vi "HCCConfig.vi"() -> ()   [LabVIEW 2014]
uses:
  c_MicroZedInstr_Enum.ctl
  g_ReportControl.vi
  <vilib>/Utility/file.llb/Read From Spreadsheet File (string).vi
  g_HCCRegisterConfig.vi
  <vilib>/Utility/file.llb/Write To Spreadsheet File (string).vi
  g_MicroZed_Interface.vi
  g_Stop.vi
  <vilib>/regexp/Match Regular Expression.xnode
panel:
  out "Transmission Error":bool
  in  "Register":T1(ring)
  in  "Write Register":bool
  in  "Value":string=" 0x00000000"
  in  "OK":bool
  out "Table":string[][](table)=[["HCC Register", "Address", "Value", "Default Values"], ["HCC_REG_0", " 0x00", "", " 0x0007FEC5"], ["HCC_REG_1", " 0x01", "", " 0xE0018080"], ["HCC_REG_2", " 0x02", "", " 0x00000840"], ["HCC_REG_3", " 0x03", "", " 0x000FFC00"], ["HCC_REG_4", " 0x04", "", " 0x3FF003FF"], ["HCC_REG_5", " 0x05", "", " 0x000FFC00"], ["HCC_REG_6", " 0x06", "", " 0x3FF003FF"], ["HCC_REG_7", " 0x07", "", " 0x000FFC00"], ["HCC_REG_8", " 0x08", "", " 0x00000000"], ["HCC_REG_9", " 0x09", "", " 0x39CE739C"], ["HCC_REG_10", " 0x10", "", " 0x00333304"], ["HCC_REG_11", " 0x11", "", " 0x01050402"], ["HCC_REG_12", " 0x12", "", " 0x00000000"], ["HCC_REG_13", " 0x13", "", " 0x00700000"], ["HCC_REG_14", " 0x14", "", " 0xFFF107FF"], ["HCC_REG_15", " 0x15", "", " 0xFFFFFFFF"], ["HCC_REG_16", " 0x16", "", " 0x00000000"], ["HCC_REG_17", " 0x17", "", " 0x00000000"]]
  in  "Store Custom":bool
  in  "Load Default":bool
  in  "Load Config File":bool
  # "HCC Register Configuration"
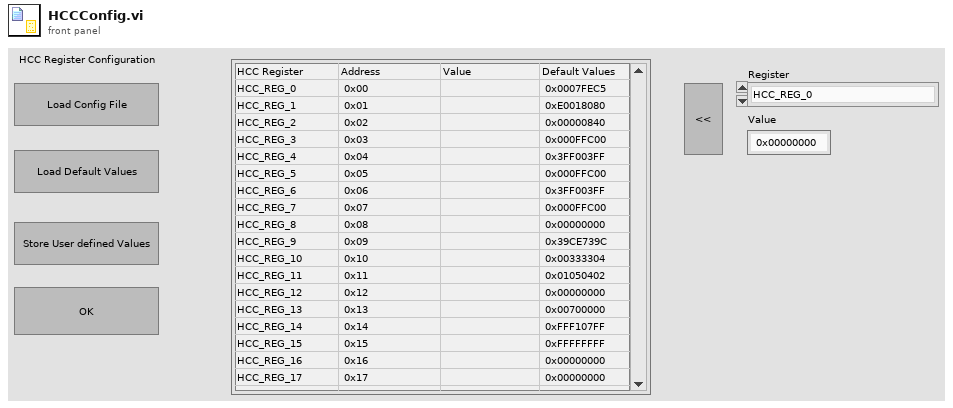
[diagram p1: front panel]
types:
  T1 = enum16{"HCC_REG_0", "HCC_REG_1", "HCC_REG_2", "HCC_REG_3", "HCC_REG_4", "HCC_REG_5", "HCC_REG_6", "HCC_REG_7", "HCC_REG_8", "HCC_REG_9", "HCC_REG_10", "HCC_REG_11", "HCC_REG_12", "HCC_REG_13", "HCC_REG_14", "HCC_REG_15", "HCC_REG_16", "HCC_REG_17"}
  T2 = typedef "c_MicroZedInstr_Enum.ctl" = enum16{"Start Test Procedure", "Print Instructions", "Config HCC Register", "Send Parameters"}
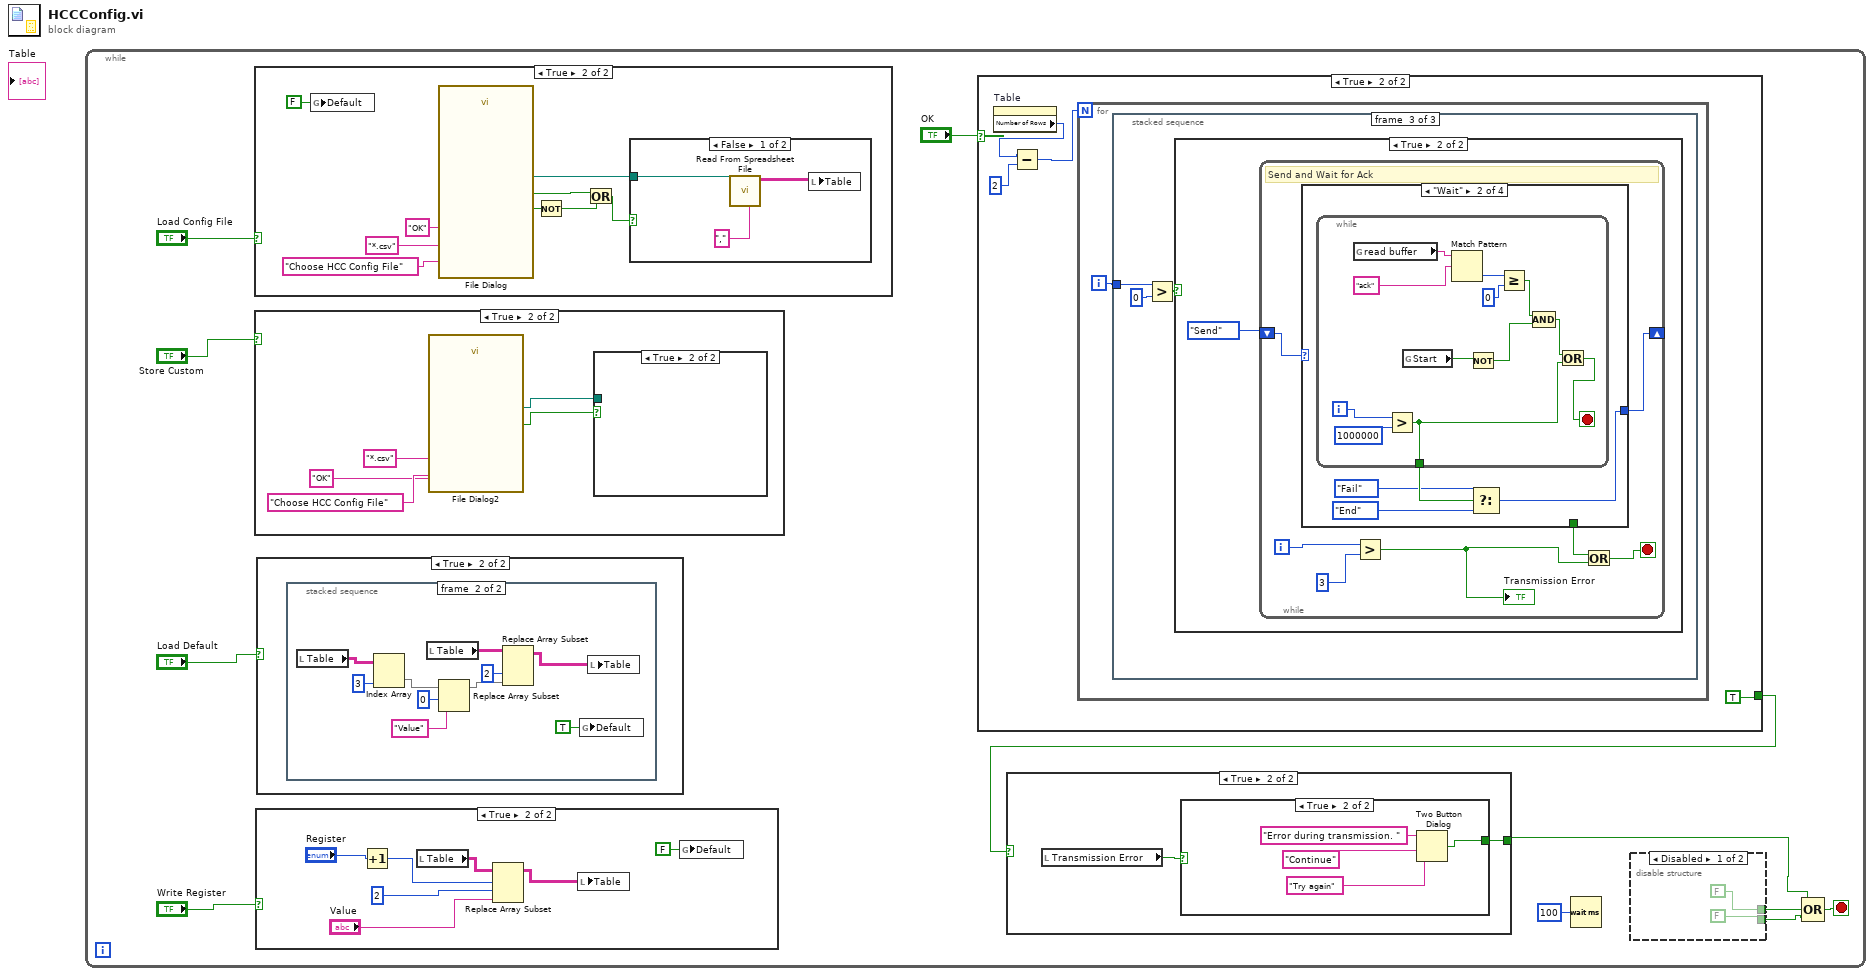
[diagram p0: block diagram]
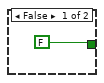
[diagram p2: hidden frame]
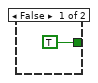
[diagram p3: hidden frame]
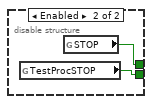
[diagram p4: hidden frame]
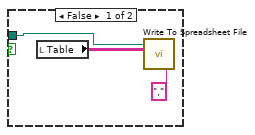
[diagram p6: hidden frame]
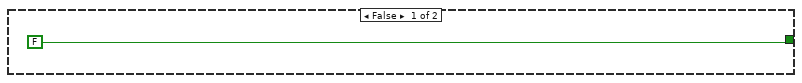
[diagram p8: hidden frame]
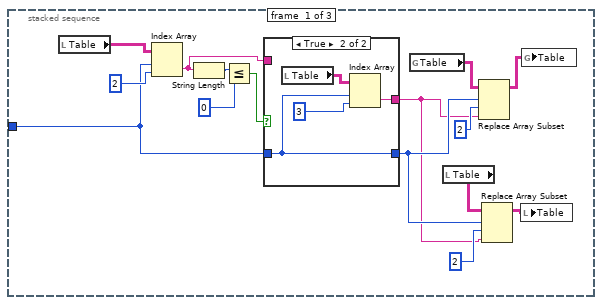
[diagram p9: hidden frame]
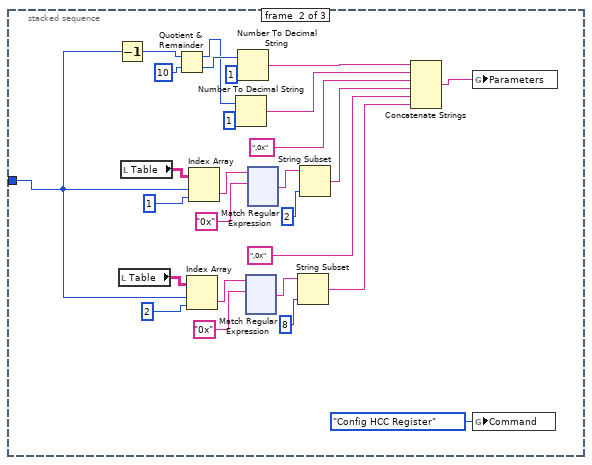
[diagram p11: hidden frame]
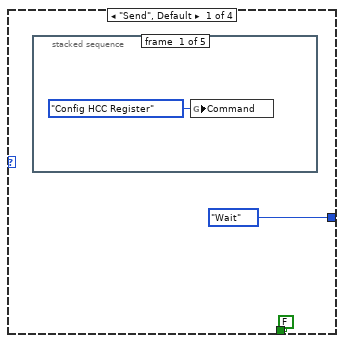
[diagram p13: hidden frame]
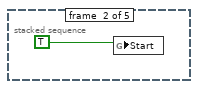
[diagram p14: hidden frame]
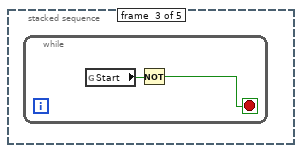
[diagram p15: hidden frame]
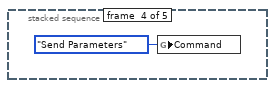
[diagram p16: hidden frame]
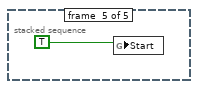
[diagram p17: hidden frame]
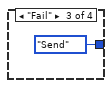
[diagram p18: hidden frame]
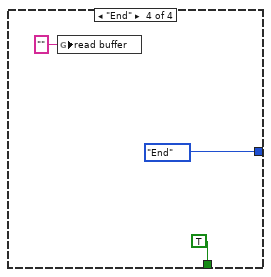
[diagram p19: hidden frame]
diagram:
  n1 = while {
    stop <- w5 stop-if-true
    n2 = case shown="True" "Load Config File" {
      frame False {
        n3 = global write "g_ReportControl.vi" "New Report"(FALSE ("New Report")) -> ()
      }
      frame True {
        n4 = global write "g_HCCRegisterConfig.vi" "Default"(FALSE ("Default")) -> ()
        n5 = call "File Dialog"("prompt"="Choose HCC Config File", "button label"="OK", "pattern (all files)"="*.csv") -> ("selected path"=w373:path, "exists"=w377:bool, "cancelled"=w375:bool)  [unwired: 9 in, 1 out]
        n6 = Not(x=w377) -> (.not. x?=w376:bool)
        n7 = Or(x=w375, y=w376) -> (x .or. y?=w374:bool)
        n8 = case shown="False" w374 {
          tunnel: w373 -> [w383 _]
          frame False {
            n9 = call-poly <vilib>:"Read From Spreadsheet File.vi"("delimiter (\\t)"="," ("delimiter (\\t)"), "file path (dialog if empty)"=w383) -> ("all rows"=w381:string[][])  [unwired: 5 in, 4 out]
            n10 = local write "Table"(w381) -> ()
          }
          frame True {
            n11 = One Button Dialog(message="Config File could not be loaded") -> ()  [unwired: 1 in, 1 out]
          }
        }
      }
    }
    n12 = case shown="True" "Store Custom" {
      frame False {
      }
      frame True {
        n13 = call "File Dialog2"("prompt"="Choose HCC Config File", "button label"="OK", "pattern (all files)"="*.csv") -> ("selected path"=w25:path, "cancelled"=w24:bool)  [unwired: 9 in, 2 out]
        n14 = case shown="True" w24 {
          tunnel: w25 -> [w29 _]
          frame False {
            n15 = local read "Table"() -> (w30:string[][])
            n16 = call-poly <vilib>:"Write To Spreadsheet File.vi"("delimiter (\\t)"="," ("delimiter (\\t)"), "2D data"=w30, "file path (dialog if empty)"=w29) -> ()  [unwired: 5 in, 1 out]
          }
          frame True {
          }
        }
      }
    }
    n17 = case shown="True" "Write Register" {
      frame False {
      }
      frame True {
        n18 = Increment(x="Register") -> (x+1=w33:T1)
        n19 = local read "Table"() -> (w37:string[][])
        n20 = Replace Array Subset(array=w37, new element="Value", index (row)=w33, index (col)=2 ("disabled index (col)")) -> (w38:string[][])
        n21 = local write "Table"(w38) -> ()
        n22 = global write "g_HCCRegisterConfig.vi" "Default"(FALSE ("Default")) -> ()
      }
    }
    n23 = case shown="True" "Load Default" {
      frame False {
      }
      frame True {
        n24 = stacked-sequence {
          frame #0 {
            n25 = control-ref of="Table"() -> (w360:refnum<vi>)
            n26 = invoke class="Tbl (strict)" method="Reinit To Default"(reference=w360) -> ()  [unwired: 2 in, 3 out]
          }
          frame #1 {
            n27 = local read "Table"() -> (w370:string[][])
            n28 = Index Array(array=w370, index (col)=3 ("disabled index (col)")) -> (element=w368:string[])  [unwired: 1 in]
            n29 = local read "Table"() -> (w364:string[][])
            n30 = Replace Array Subset(array=w368, new element="Value" ("new element/subarray"), index=0) -> (w365:string[])
            n31 = Replace Array Subset(array=w364, new element=w365, index (col)=2 ("disabled index (col)")) -> (w362:string[][])  [unwired: 1 in]
            n32 = global write "g_HCCRegisterConfig.vi" "Default"(TRUE ("Default")) -> ()
            n33 = local write "Table"(w362) -> ()
          }
        }
      }
    }
    n34 = case shown="True" "OK" {
      tunnel: [FALSE TRUE] -> w2
      frame False {
      }
      frame True {
        n35 = property on="Table" class="Tbl (strict)"() -> ("Number of Rows"=w42:u32)  [unwired: 2 in, 2 out]
        n36 = Subtract(x=w42, y=u32 2) -> (x-y=w41:u32)
        n37 = for {
          N: w41 -> [_]
          i -> [w44]
          n38 = stacked-sequence {
            tunnel: w44 -> [w50 w66 w323]
            frame #0 {
              n39 = local read "Table"() -> (w52:string[][])
              n40 = Index Array(array=w52, index (row)=w50, index (col)=2 ("disabled index (col)")) -> (element=w51:string)
              n41 = String Length(string=w51) -> (length=w58:i32)
              n42 = Less Or Equal?(x=w58, y=0) -> (x <= y?=w56:bool)
              n43 = case shown="True" w56 {
                tunnel: w50 -> [w61 w63]
                tunnel: [w61 w63] -> w46
                tunnel: [w60 w62] -> w45
                tunnel: w51 -> [w60 _]
                frame False {
                }
                frame True {
                  n44 = local read "Table"() -> (w64:string[][])
                  n45 = Index Array(array=w64, index (row)=w63, index (col)=3 ("disabled index (col)")) -> (element=w62:string)
                }
              }
              n46 = global read "g_HCCRegisterConfig.vi" "Table"() -> (w55:string[][])
              n47 = local read "Table"() -> (w48:string[][])
              n48 = Replace Array Subset(array=w55, new element=w45, index (row)=w46, index (col)=2 ("disabled index (col)")) -> (w54:string[][])
              n49 = Replace Array Subset(array=w48, new element=w45, index (row)=w46, index (col)=2 ("disabled index (col)")) -> (w47:string[][])
              n50 = local write "Table"(w47) -> ()
              n51 = global write "g_HCCRegisterConfig.vi" "Table"(w54) -> ()
            }
            frame #1 {
              n52 = Decrement(x=w66) -> (x-1=w67:i32)
              n53 = local read "Table"() -> (w80:string[][])
              n54 = local read "Table"() -> (w89:string[][])
              n55 = Quotient & Remainder(x=w67, y=10) -> (x-y*floor(x/y)=w68:i32, floor(x/y)=w69:i32)
              n56 = Index Array(array=w80, index (row)=w66, index (col)=2 ("disabled index (col)")) -> (element=w82:string)
              n57 = Index Array(array=w89, index (row)=w66, index (col)=1 ("disabled index (col)")) -> (element=w87:string)
              n58 = Number To Decimal String(number=w68, width (-)=i16 1) -> (decimal integer string=w77:string)
              n59 = Number To Decimal String(number=w69, width (-)=i16 1) -> (decimal integer string=w79:string)
              n60 = xnode ("Match Regular Expression")("input string"=w82, "regular expression"="0x") -> ("after match"=w70:string)  [unwired: 4 in, 4 out]
              n61 = xnode ("Match Regular Expression")("input string"=w87, "regular expression"="0x") -> ("after match"=w71:string)  [unwired: 4 in, 4 out]
              n62 = String Subset(string=w70, length (rest)=8 ("length (rest)")) -> (substring=w73:string)  [unwired: 1 in]
              n63 = String Subset(string=w71, length (rest)=2 ("length (rest)")) -> (substring=w75:string)  [unwired: 1 in]
              n64 = Concatenate Strings(w79, w77, ",0x", w75, ",0x", w73) -> (w78:string)
              n65 = global write "g_MicroZed_Interface.vi" "Parameters"(w78) -> ()
              n66 = global write "g_MicroZed_Interface.vi" "Command"(c_MicroZedInstr_Enum."Config HCC Register" ("Command")) -> ()
            }
            frame #2 {
              n67 = Greater?(x=w323, y=0) -> (0:w321:bool)
              n68 = case shown="True" w321 {
                frame False {
                }
                frame True {
                  n69 = while {
                    shift-right: [w330] -> _
                    shift-left: enum16{"Send", "Wait", "Fail", "End"}."Send" -> [w331]
                    i -> [w329]
                    stop <- w327 stop-if-true
                    # "Send and Wait for Ack"
                    n70 = case shown="\"Wait\"" w331 {
                      tunnel: [enum16{"Send", "Wait", "Fail"}."Wait" w340 enum16{"Send", "Wait", "Fail"}."Send" enum16{"Send", "Wait", "Fail", "End"}."End"] -> w330
                      tunnel: [FALSE _ _ TRUE] -> w326
                      frame "Send", Default {
                        n71 = stacked-sequence {
                          frame #0 {
                            n72 = global write "g_MicroZed_Interface.vi" "Command"(c_MicroZedInstr_Enum."Config HCC Register" ("Command")) -> ()
                          }
                          frame #1 {
                            n73 = global write "g_MicroZed_Interface.vi" "Start"(TRUE ("Start")) -> ()
                          }
                          frame #2 {
                            n74 = while {
                              stop <- w336 stop-if-true
                              n75 = global read "g_MicroZed_Interface.vi" "Start"() -> (w337:bool)
                              n76 = Not(x=w337) -> (.not. x?=w336:bool)
                            }
                          }
                          frame #3 {
                            n77 = global write "g_MicroZed_Interface.vi" "Command"(c_MicroZedInstr_Enum."Send Parameters" ("Command")) -> ()
                          }
                          frame #4 {
                            n78 = global write "g_MicroZed_Interface.vi" "Start"(TRUE ("Start")) -> ()
                          }
                        }
                      }
                      frame "Wait" {
                        n79 = while {
                          tunnel: [w344] -> w343
                          i -> [w348]
                          stop <- w346 stop-if-true
                          n80 = global read "g_MicroZed_Interface.vi" "read buffer"() -> (w352:string)
                          n81 = Greater?(x=w348, y=1000000) -> (0:w344:bool)
                          n82 = global read "g_MicroZed_Interface.vi" "Start"() -> (w355:bool)
                          n83 = Match Pattern(string=w352, regular expression="ack" ("y")) -> (offset past match=w350:i32)  [unwired: 1 in, 3 out]
                          n84 = Not(x=w355) -> (.not. x?=w353:bool)
                          n85 = Greater Or Equal?(x=w350, y=0) -> (x >= y?=w354:bool)
                          n86 = Compound Arithmetic op=AND(w354, w353) -> (w345:bool)
                          n87 = Or(x=w345, y=w344) -> (x .or. y?=w346:bool)
                        }
                        n88 = Select(t=enum16{"Send", "Wait", "Fail", "End"}."Fail", s=w343, f=enum16{"Send", "Wait", "Fail", "End"}."End") -> (s? t:f=w340:enum16{"Send", "Wait", "Fail", "End"})
                      }
                      frame "Fail" {
                      }
                      frame "End" {
                        n89 = global write "g_MicroZed_Interface.vi" "read buffer"("" ("read buffer")) -> ()
                      }
                    }
                    n90 = Greater?(x=w329, y=3) -> (0:w325:bool)
                    "Transmission Error" <- w325
                    n91 = Or(x=w326, y=w325) -> (x .or. y?=w327:bool)
                  }
                }
              }
            }
          }
        }
      }
    }
    n92 = case shown="True" w2 {
      tunnel: [FALSE w13] -> w1
      frame False {
      }
      frame True {
        n93 = local read "Transmission Error"() -> (w14:bool)
        n94 = case shown="True" w14 {
          tunnel: [TRUE w19] -> w13
          frame False {
          }
          frame True {
            n95 = Two Button Dialog(message="Error during transmission. ", 1:"Try again" ("F button name (\"Cancel\")"), 2:"Continue" ("T button name (\"OK\")")) -> (T button?=w19:bool)
          }
        }
      }
    }
    n96 = Wait (ms)(milliseconds to wait=u32 100) -> ()  [unwired: 1 out]
    n97 = disable-structure shown="Disabled" {
      disable-tunnel: [FALSE w23] -> w4
      disable-tunnel: [FALSE w22] -> w3
      frame Disabled {
      }
      frame Enabled {
        n98 = global read "g_Stop.vi" "TestProcSTOP"() -> (w22:bool)
        n99 = global read "g_Stop.vi" "STOP"() -> (w23:bool)
      }
    }
    n100 = Compound Arithmetic op=OR(w1, w4, w3) -> (w5:bool)
  }
